vi "Dynamic Headers Change Headers.vi"(6 "Point Startup (WasherDOE)":path, 7 "Tree Selection":T2="1-1", 8 "Error In":errorcluster, 10 "Tool Base Path":path=path "C:/Technology Lab/NI-2010/Trunk/Refrigeration/RTS/Old System", 11 "Chamber Data":string[][](array[string])=[["System Date", "System Time", "Elapsed Time (sec)", "Elapsed Time (hrs)", "Voltage (V)", "RMS Current (Amps)", "Power (Watts)", "Watt Hours (Wh)", "Voltage Total Harmonic Distortion (%)", "Frequency (Hz)", "Apparent Power (VA)", "Power Factor", "TC 1", "TC 2", "TC 3", "TC 4", "TC 5", "TC 6", "TC 7", "TC 8", "TC 9", "TC 10", "TC 11", "TC 12", "TC 13", "TC 14", "TC 15", "TC 16", "TC 17", "TC 18", "TC 19", "TC 20", "TC 21", "TC 22", "TC 23", "TC 24", "TC 25", "TC 26", "TC 27", "TC 28", "TC 29", "TC 30", "AUX 1", "AUX 2", "CAL CL", "Room Setpoint Temperature", "Room Setpoint Humidity", "Room Temperature (°F)", "Room Humidity (%)", "Door Enable", "Room Setpoint Cool Temperature", "Room Setpoint Dehumidification Temperature", "Supply Temperature (°F)", "Cool Temperature (°F)", "Dehumidification Temperature (°F)", "Glycol Temperature (°F)", "Heat Rate (%)", "Steam Rate (%)", "Cool Rate (%)", "Dehumidification Rate (%)", "Room Status", "Room Dry P", "Room Dry I", "Room Humidity P", "Room Humidity I", "Room Heat P", "Room Heat I", "Room Cool Temperature P", "Room Cool Temperature I", "Room Dehumidification Temperature P", "Room Dehumidification Temperature I", "Voltage Setpoint 1", "60 Hz Power", "50 Hz Power", "120V Range", "240V Range", "Ground Line", "Ground Neutral", "Measure Ground Leakage Current", "Room OK", "S1 Freezer Relay", "S1 Cab Relay", "S1 Slide Relay", "Recording Data", "CVS Location", "Point Location"], ["01/24/2018", "06:36:24.375", "0.000000", "0.000000", "115.046623", "0.030182", "0.135573", "964.507616", "3.000000", "60.021709", "3.472371", "1.000000", "-2.310000", "-1.920000", "-0.910000", "327.670000", "327.670000", "327.670000", "327.670000", "327.670000", "327.670000", "327.670000", "38.020000", "35.660000", "35.030000", "327.670000", "327.670000", "327.670000", "327.670000", "327.670000", "327.670000", "327.670000", "327.670000", "327.670000", "327.670000", "70.360000", "327.670000", "327.670000", "70.300000", "327.670000", "32767.000000", "32767.000000", "0.001000", "0.000000", "1.988000", "70.000000", "35.000000", "70.040000", "38.150000", "1.000000", "55.000000", "48.000000", "66.700000", "55.180000", "48.160000", "0.000000", "36.920000", "0.000000", "30.630000", "8.240000", "0.000000", "200.000000", "15000.000000", "400.000000", "15000.000000", "1000.000000", "2000.000000", "500.000000", "6000.000000", "500.000000", "6000.000000", "115.000000", "1.000000", "0.000000", "1.000000", "0.000000", "0.000000", "1.000000", "0.000000", "1.000000", "0.000000", "0.000000", "0.000000", "FALSE", "", ""], ["System Date", "System Time", "Elapsed Time (sec)", "Elapsed Time (hrs)", "Voltage (V)", "RMS Current (Amps)", "Power (Watts)", "Watt Hours (Wh)", "Voltage Total Harmonic Distortion (%)", "Frequency (Hz)", "Apparent Power (VA)", "Power Factor", "TC 1", "TC 2", "TC 3", "TC 4", "TC 5", "TC 6", "TC 7", "TC 8", "TC 9", "TC 10", "TC 11", "TC 12", "TC 13", "TC 14", "TC 15", "TC 16", "TC 17", "TC 18", "TC 19", "TC 20", "TC 21", "TC 22", "TC 23", "TC 24", "TC 25", "TC 26", "TC 27", "TC 28", "TC 29", "TC 30", "AUX 1", "AUX 2", "CAL CL", "Room Setpoint Temperature", "Room Setpoint Humidity", "Room Temperature (°F)", "Room Humidity (%)", "Door Enable", "Room Setpoint Cool Temperature", "Room Setpoint Dehumidification Temperature", "Supply Temperature (°F)", "Cool Temperature (°F)", "Dehumidification Temperature (°F)", "Glycol Temperature (°F)", "Heat Rate (%)", "Steam Rate (%)", "Cool Rate (%)", "Dehumidification Rate (%)", "Room Status", "Room Dry P", "Room Dry I", "Room Humidity P", "Room Humidity I", "Room Heat P", "Room Heat I", "Room Cool Temperature P", "Room Cool Temperature I", "Room Dehumidification Temperature P", "Room Dehumidification Temperature I", "Voltage Setpoint 2", "60 Hz Power", "50 Hz Power", "120V Range", "240V Range", "Ground Line", "Ground Neutral", "Measure Ground Leakage Current", "Fault", "S2 Freezer Relay", "S2 Cab Relay", "S2 Slide Relay", "Recording Data", "CVS Location", "Point Location"], ["01/24/2018", "06:36:24.375", "0.000000", "0.000000", "114.863785", "0.030740", "0.139474", "26203.680290", "3.500000", "60.021633", "3.530865", "1.000000", "10.000000", "8.600000", "8.210000", "327.670000", "327.670000", "327.670000", "327.670000", "327.670000", "327.670000", "327.670000", "41.900000", "42.090000", "43.130000", "327.670000", "327.670000", "327.670000", "327.670000", "327.670000", "327.670000", "327.670000", "327.670000", "327.670000", "327.670000", "69.920000", "327.670000", "327.670000", "70.410000", "327.670000", "32767.000000", "32767.000000", "0.001000", "0.001000", "1.991000", "70.000000", "35.000000", "70.040000", "38.150000", "1.000000", "55.000000", "48.000000", "66.700000", "55.180000", "48.160000", "0.000000", "36.920000", "0.000000", "30.630000", "8.240000", "0.000000", "200.000000", "15000.000000", "400.000000", "15000.000000", "1000.000000", "2000.000000", "500.000000", "6000.000000", "500.000000", "6000.000000", "115.000000", "1.000000", "0.000000", "1.000000", "0.000000", "0.000000", "1.000000", "0.000000", "0.000000", "0.000000", "0.000000", "0.000000", "FALSE", "", ""], ["System Date", "System Time", "Elapsed Time (sec)", "Elapsed Time (hrs)", "Voltage (V)", "RMS Current (Amps)", "Power (Watts)", "Watt Hours (Wh)", "Voltage Total Harmonic Distortion (%)", "Frequency (Hz)", "Apparent Power (VA)", "Power Factor", "TC 1", "TC 2", "TC 3", "TC 4", "TC 5", "TC 6", "TC 7", "TC 8", "TC 9", "TC 10", "TC 11", "TC 12", "TC 13", "TC 14", "TC 15", "TC 16", "TC 17", "TC 18", "TC 19", "TC 20", "TC 21", "TC 22", "TC 23", "TC 24", "TC 25", "TC 26", "TC 27", "TC 28", "TC 29", "TC 30", "AUX 1", "AUX 2", "CAL CL", "Room Setpoint Temperature", "Room Setpoint Humidity", "Room Temperature (°F)", "Room Humidity (%)", "Door Enable", "Room Setpoint Cool Temperature", "Room Setpoint Dehumidification Temperature", "Supply Temperature (°F)", "Cool Temperature (°F)", "Dehumidification Temperature (°F)", "Glycol Temperature (°F)", "Heat Rate (%)", "Steam Rate (%)", "Cool Rate (%)", "Dehumidification Rate (%)", "Room Status", "Room Dry P", "Room Dry I", "Room Humidity P", "Room Humidity I", "Room Heat P", "Room Heat I", "Room Cool Temperature P", "Room Cool Temperature I", "Room Dehumidification Temperature P", "Room Dehumidification Temperature I", "Voltage Setpoint 3", "60 Hz Power", "50 Hz Power", "120V Range", "240V Range", "Ground Line", "Ground Neutral", "Measure Ground Leakage Current", "Room Heat", "S3 Freezer Relay", "S3 Cab Relay", "S3 Slide Relay", "Recording Data", "CVS Location", "Point Location"], ["01/24/2018", "06:36:24.376", "0.000000", "0.000000", "114.844543", "0.030078", "0.135316", "27955.201782", "3.100000", "60.022556", "3.456682", "1.000000", "0.690000", "0.850000", "2.060000", "327.670000", "327.670000", "327.670000", "327.670000", "327.670000", "327.670000", "327.670000", "37.750000", "38.160000", "38.080000", "327.670000", "327.670000", "327.670000", "327.670000", "327.670000", "327.670000", "327.670000", "327.670000", "327.670000", "327.670000", "70.410000", "327.670000", "327.670000", "70.770000", "327.670000", "32767.000000", "32767.000000", "0.001000", "0.001000", "1.963000", "70.000000", "35.000000", "70.040000", "38.150000", "1.000000", "55.000000", "48.000000", "66.700000", "55.180000", "48.160000", "0.000000", "36.920000", "0.000000", "30.630000", "8.240000", "0.000000", "200.000000", "15000.000000", "400.000000", "15000.000000", "1000.000000", "2000.000000", "500.000000", "6000.000000", "500.000000", "6000.000000", "115.000000", "1.000000", "0.000000", "1.000000", "0.000000", "0.000000", "1.000000", "0.000000", "1.000000", "0.000000", "0.000000", "0.000000", "FALSE", "", ""], ["System Date", "System Time", "Elapsed Time (sec)", "Elapsed Time (hrs)", "Voltage (V)", "RMS Current (Amps)", "Power (Watts)", "Watt Hours (Wh)", "Voltage Total Harmonic Distortion (%)", "Frequency (Hz)", "Apparent Power (VA)", "Power Factor", "TC 1", "TC 2", "TC 3", "TC 4", "TC 5", "TC 6", "TC 7", "TC 8", "TC 9", "TC 10", "TC 11", "TC 12", "TC 13", "TC 14", "TC 15", "TC 16", "TC 17", "TC 18", "TC 19", "TC 20", "TC 21", "TC 22", "TC 23", "TC 24", "TC 25", "TC 26", "TC 27", "TC 28", "TC 29", "TC 30", "AUX 1", "AUX 2", "CAL CL", "Room Setpoint Temperature", "Room Setpoint Humidity", "Room Temperature (°F)", "Room Humidity (%)", "Door Enable", "Room Setpoint Cool Temperature", "Room Setpoint Dehumidification Temperature", "Supply Temperature (°F)", "Cool Temperature (°F)", "Dehumidification Temperature (°F)", "Glycol Temperature (°F)", "Heat Rate (%)", "Steam Rate (%)", "Cool Rate (%)", "Dehumidification Rate (%)", "Room Status", "Room Dry P", "Room Dry I", "Room Humidity P", "Room Humidity I", "Room Heat P", "Room Heat I", "Room Cool Temperature P", "Room Cool Temperature I", "Room Dehumidification Temperature P", "Room Dehumidification Temperature I", "Voltage Setpoint 4", "60 Hz Power", "50 Hz Power", "120V Range", "240V Range", "Ground Line", "Ground Neutral", "Measure Ground Leakage Current", "Room Blower", "S4 Freezer Relay", "S4 Cab Relay", "S4 Slide Relay", "Recording Data", "CVS Location", "Point Location"], ["01/24/2018", "06:36:24.376", "0.000000", "0.000000", "115.200577", "0.030417", "0.136655", "26339.492026", "3.200000", "60.021862", "3.504017", "1.000000", "1.700000", "3.490000", "4.180000", "327.670000", "327.670000", "327.670000", "327.670000", "327.670000", "327.670000", "327.670000", "38.630000", "39.700000", "39.970000", "327.670000", "327.670000", "327.670000", "327.670000", "327.670000", "327.670000", "327.670000", "327.670000", "327.670000", "327.670000", "70.410000", "327.670000", "327.670000", "70.880000", "327.670000", "32767.000000", "32767.000000", "0.001000", "0.000000", "2.005000", "70.000000", "35.000000", "70.040000", "38.150000", "1.000000", "55.000000", "48.000000", "66.700000", "55.180000", "48.160000", "0.000000", "36.920000", "0.000000", "30.630000", "8.240000", "0.000000", "200.000000", "15000.000000", "400.000000", "15000.000000", "1000.000000", "2000.000000", "500.000000", "6000.000000", "500.000000", "6000.000000", "115.000000", "1.000000", "0.000000", "1.000000", "0.000000", "0.000000", "1.000000", "0.000000", "1.000000", "0.000000", "0.000000", "0.000000", "FALSE", "", ""], ["System Date", "System Time", "Elapsed Time (sec)", "Elapsed Time (hrs)", "Voltage (V)", "RMS Current (Amps)", "Power (Watts)", "Watt Hours (Wh)", "Voltage Total Harmonic Distortion (%)", "Frequency (Hz)", "Apparent Power (VA)", "Power Factor", "TC 1", "TC 2", "TC 3", "TC 4", "TC 5", "TC 6", "TC 7", "TC 8", "TC 9", "TC 10", "TC 11", "TC 12", "TC 13", "TC 14", "TC 15", "TC 16", "TC 17", "TC 18", "TC 19", "TC 20", "TC 21", "TC 22", "TC 23", "TC 24", "TC 25", "TC 26", "TC 27", "TC 28", "TC 29", "TC 30", "AUX 1", "AUX 2", "CAL CL", "Room Setpoint Temperature", "Room Setpoint Humidity", "Room Temperature (°F)", "Room Humidity (%)", "Door Enable", "Room Setpoint Cool Temperature", "Room Setpoint Dehumidification Temperature", "Supply Temperature (°F)", "Cool Temperature (°F)", "Dehumidification Temperature (°F)", "Glycol Temperature (°F)", "Heat Rate (%)", "Steam Rate (%)", "Cool Rate (%)", "Dehumidification Rate (%)", "Room Status", "Room Dry P", "Room Dry I", "Room Humidity P", "Room Humidity I", "Room Heat P", "Room Heat I", "Room Cool Temperature P", "Room Cool Temperature I", "Room Dehumidification Temperature P", "Room Dehumidification Temperature I", "Voltage Setpoint 5", "60 Hz Power", "50 Hz Power", "120V Range", "240V Range", "Ground Line", "Ground Neutral", "Measure Ground Leakage Current", "Spare", "S5 Freezer Relay", "S5 Cab Relay", "S5 Slide Relay", "Recording Data", "CVS Location", "Point Location"], ["01/24/2018", "06:36:24.376", "0.000000", "0.000000", "115.123596", "0.000000", "0.000000", "0.000000", "3.300000", "60.022747", "0.000000", "1.000000", "327.670000", "327.670000", "70.410000", "327.670000", "327.670000", "327.670000", "327.670000", "327.670000", "327.670000", "327.670000", "70.630000", "70.360000", "70.360000", "327.670000", "327.670000", "327.670000", "327.670000", "327.670000", "327.670000", "327.670000", "327.670000", "327.670000", "327.670000", "69.950000", "327.670000", "327.670000", "327.670000", "327.670000", "32767.000000", "32767.000000", "0.001000", "0.001000", "1.999000", "70.000000", "35.000000", "70.040000", "38.150000", "1.000000", "55.000000", "48.000000", "66.700000", "55.180000", "48.160000", "0.000000", "36.920000", "0.000000", "30.630000", "8.240000", "0.000000", "200.000000", "15000.000000", "400.000000", "15000.000000", "1000.000000", "2000.000000", "500.000000", "6000.000000", "500.000000", "6000.000000", "115.000000", "1.000000", "0.000000", "1.000000", "0.000000", "0.000000", "1.000000", "0.000000", "0.000000", "0.000000", "0.000000", "0.000000", "FALSE", "", ""], ["System Date", "System Time", "Elapsed Time (sec)", "Elapsed Time (hrs)", "Voltage (V)", "RMS Current (Amps)", "Power (Watts)", "Watt Hours (Wh)", "Voltage Total Harmonic Distortion (%)", "Frequency (Hz)", "Apparent Power (VA)", "Power Factor", "TC 1", "TC 2", "TC 3", "TC 4", "TC 5", "TC 6", "TC 7", "TC 8", "TC 9", "TC 10", "TC 11", "TC 12", "TC 13", "TC 14", "TC 15", "TC 16", "TC 17", "TC 18", "TC 19", "TC 20", "TC 21", "TC 22", "TC 23", "TC 24", "TC 25", "TC 26", "TC 27", "TC 28", "TC 29", "TC 30", "AUX 1", "AUX 2", "CAL CL", "Room Setpoint Temperature", "Room Setpoint Humidity", "Room Temperature (°F)", "Room Humidity (%)", "Door Enable", "Room Setpoint Cool Temperature", "Room Setpoint Dehumidification Temperature", "Supply Temperature (°F)", "Cool Temperature (°F)", "Dehumidification Temperature (°F)", "Glycol Temperature (°F)", "Heat Rate (%)", "Steam Rate (%)", "Cool Rate (%)", "Dehumidification Rate (%)", "Room Status", "Room Dry P", "Room Dry I", "Room Humidity P", "Room Humidity I", "Room Heat P", "Room Heat I", "Room Cool Temperature P", "Room Cool Temperature I", "Room Dehumidification Temperature P", "Room Dehumidification Temperature I", "Voltage Setpoint 6", "60 Hz Power", "50 Hz Power", "120V Range", "240V Range", "Ground Line", "Ground Neutral", "Measure Ground Leakage Current", "Room Pump", "S6 Freezer Relay", "S6 Cab Relay", "S6 Slide Relay", "Recording Data", "CVS Location", "Point Location"], ["01/24/2018", "06:36:24.376", "0.000000", "0.000000", "114.825302", "0.000000", "0.000000", "0.000000", "3.400000", "60.022854", "0.000000", "1.000000", "327.670000", "327.670000", "327.670000", "327.670000", "327.670000", "327.670000", "327.670000", "327.670000", "327.670000", "327.670000", "327.670000", "327.670000", "327.670000", "327.670000", "327.670000", "327.670000", "327.670000", "327.670000", "327.670000", "327.670000", "327.670000", "327.670000", "327.670000", "327.670000", "327.670000", "327.670000", "327.670000", "327.670000", "32767.000000", "32767.000000", "0.001000", "0.001000", "1.995000", "70.000000", "35.000000", "70.040000", "38.150000", "1.000000", "55.000000", "48.000000", "66.700000", "55.180000", "48.160000", "0.000000", "36.920000", "0.000000", "30.630000", "8.240000", "0.000000", "200.000000", "15000.000000", "400.000000", "15000.000000", "1000.000000", "2000.000000", "500.000000", "6000.000000", "500.000000", "6000.000000", "115.000000", "1.000000", "0.000000", "1.000000", "0.000000", "0.000000", "1.000000", "0.000000", "1.000000", "0.000000", "0.000000", "0.000000", "FALSE", "", ""], ["System Date", "System Time", "Elapsed Time (sec)", "Elapsed Time (hrs)", "Voltage (V)", "RMS Current (Amps)", "Power (Watts)", "Watt Hours (Wh)", "Voltage Total Harmonic Distortion (%)", "Frequency (Hz)", "Apparent Power (VA)", "Power Factor", "TC 1", "TC 2", "TC 3", "TC 4", "TC 5", "TC 6", "TC 7", "TC 8", "TC 9", "TC 10", "TC 11", "TC 12", "TC 13", "TC 14", "TC 15", "TC 16", "TC 17", "TC 18", "TC 19", "TC 20", "TC 21", "TC 22", "TC 23", "TC 24", "TC 25", "TC 26", "TC 27", "TC 28", "TC 29", "TC 30", "AUX 1", "AUX 2", "CAL CL", "Room Setpoint Temperature", "Room Setpoint Humidity", "Room Temperature (°F)", "Room Humidity (%)", "Door Enable", "Room Setpoint Cool Temperature", "Room Setpoint Dehumidification Temperature", "Supply Temperature (°F)", "Cool Temperature (°F)", "Dehumidification Temperature (°F)", "Glycol Temperature (°F)", "Heat Rate (%)", "Steam Rate (%)", "Cool Rate (%)", "Dehumidification Rate (%)", "Room Status", "Room Dry P", "Room Dry I", "Room Humidity P", "Room Humidity I", "Room Heat P", "Room Heat I", "Room Cool Temperature P", "Room Cool Temperature I", "Room Dehumidification Temperature P", "Room Dehumidification Temperature I", "Voltage Setpoint 7", "60 Hz Power", "50 Hz Power", "120V Range", "240V Range", "Ground Line", "Ground Neutral", "Measure Ground Leakage Current", "Spare", "S7 Freezer Relay", "S7 Cab Relay", "S7 Slide Relay", "Recording Data", "CVS Location", "Point Location"], ["01/24/2018", "06:36:24.376", "0.000000", "0.000000", "114.796432", "0.000000", "0.000000", "0.000000", "3.500000", "60.023220", "0.000000", "1.000000", "70.630000", "70.630000", "70.630000", "327.670000", "327.670000", "327.670000", "327.670000", "327.670000", "327.670000", "327.670000", "327.670000", "70.300000", "70.300000", "327.670000", "327.670000", "327.670000", "327.670000", "327.670000", "327.670000", "327.670000", "327.670000", "327.670000", "327.670000", "327.670000", "327.670000", "327.670000", "327.670000", "327.670000", "32767.000000", "32767.000000", "0.000000", "0.000000", "2.003000", "70.000000", "35.000000", "70.040000", "38.150000", "1.000000", "55.000000", "48.000000", "66.700000", "55.180000", "48.160000", "0.000000", "36.920000", "0.000000", "30.630000", "8.240000", "0.000000", "200.000000", "15000.000000", "400.000000", "15000.000000", "1000.000000", "2000.000000", "500.000000", "6000.000000", "500.000000", "6000.000000", "115.000000", "1.000000", "0.000000", "1.000000", "0.000000", "0.000000", "1.000000", "0.000000", "0.000000", "0.000000", "0.000000", "0.000000", "FALSE", "", ""], ["System Date", "System Time", "Elapsed Time (sec)", "Elapsed Time (hrs)", "Voltage (V)", "RMS Current (Amps)", "Power (Watts)", "Watt Hours (Wh)", "Voltage Total Harmonic Distortion (%)", "Frequency (Hz)", "Apparent Power (VA)", "Power Factor", "TC 1", "TC 2", "TC 3", "TC 4", "TC 5", "TC 6", "TC 7", "TC 8", "TC 9", "TC 10", "TC 11", "TC 12", "TC 13", "TC 14", "TC 15", "TC 16", "TC 17", "TC 18", "TC 19", "TC 20", "TC 21", "TC 22", "TC 23", "TC 24", "TC 25", "TC 26", "TC 27", "TC 28", "TC 29", "TC 30", "AUX 1", "AUX 2", "CAL CL", "Room Setpoint Temperature", "Room Setpoint Humidity", "Room Temperature (°F)", "Room Humidity (%)", "Door Enable", "Room Setpoint Cool Temperature", "Room Setpoint Dehumidification Temperature", "Supply Temperature (°F)", "Cool Temperature (°F)", "Dehumidification Temperature (°F)", "Glycol Temperature (°F)", "Heat Rate (%)", "Steam Rate (%)", "Cool Rate (%)", "Dehumidification Rate (%)", "Room Status", "Room Dry P", "Room Dry I", "Room Humidity P", "Room Humidity I", "Room Heat P", "Room Heat I", "Room Cool Temperature P", "Room Cool Temperature I", "Room Dehumidification Temperature P", "Room Dehumidification Temperature I", "Voltage Setpoint 8", "60 Hz Power", "50 Hz Power", "120V Range", "240V Range", "Ground Line", "Ground Neutral", "Measure Ground Leakage Current", "Spare", "S8 Freezer Relay", "S8 Cab Relay", "S8 Slide Relay", "Recording Data", "CVS Location", "Point Location"], ["01/24/2018", "06:36:24.377", "0.000000", "0.000000", "115.306419", "0.000000", "0.000000", "0.000000", "3.500000", "60.021893", "0.000000", "1.000000", "70.630000", "70.440000", "70.490000", "327.670000", "327.670000", "327.670000", "327.670000", "327.670000", "327.670000", "327.670000", "70.630000", "70.410000", "70.300000", "327.670000", "327.670000", "327.670000", "327.670000", "327.670000", "327.670000", "327.670000", "327.670000", "327.670000", "327.670000", "327.670000", "327.670000", "327.670000", "327.670000", "327.670000", "32767.000000", "32767.000000", "0.000000", "0.000000", "1.955000", "70.000000", "35.000000", "70.040000", "38.150000", "1.000000", "55.000000", "48.000000", "66.700000", "55.180000", "48.160000", "0.000000", "36.920000", "0.000000", "30.630000", "8.240000", "0.000000", "200.000000", "15000.000000", "400.000000", "15000.000000", "1000.000000", "2000.000000", "500.000000", "6000.000000", "500.000000", "6000.000000", "115.000000", "1.000000", "0.000000", "1.000000", "0.000000", "0.000000", "1.000000", "0.000000", "0.000000", "0.000000", "0.000000", "0.000000", "FALSE", "", ""]]) -> (0 "Error Out":errorcluster, 2 "Point File Path":path, 3 "New Header Save Array":T1[](array[typedef]), 5 "Default Headers":bool)   [LabVIEW 2018]
uses:
  Washer DOE/Type Definitions/DOE Data Save Modifier.ctl
  Refrigeration/RTS/Type Definitions/RTS Point File.ctl
  Refrigeration/RTS/Type Definitions/RTS Room Selector.ctl
panel:
  in  "Save Point File":bool
  in  "Delete Point File":bool
  in  "Header Save Array":T1[](array[typedef])
  in  "Point File Name":string(combo)
  in  "Use Default Headers":bool
  in  "Tab Control":enum32{"Page 1", "Page 2"}(tab)
  out "Point Data":T3[](array[typedef])
  in  "Debug":bool
  out "Debug States":string[](array[string])
  in  "Update Server":bool
  out "Front Program Name":string
  # "Name"
  # "Title"
  # "Group"
  # "Save Status"
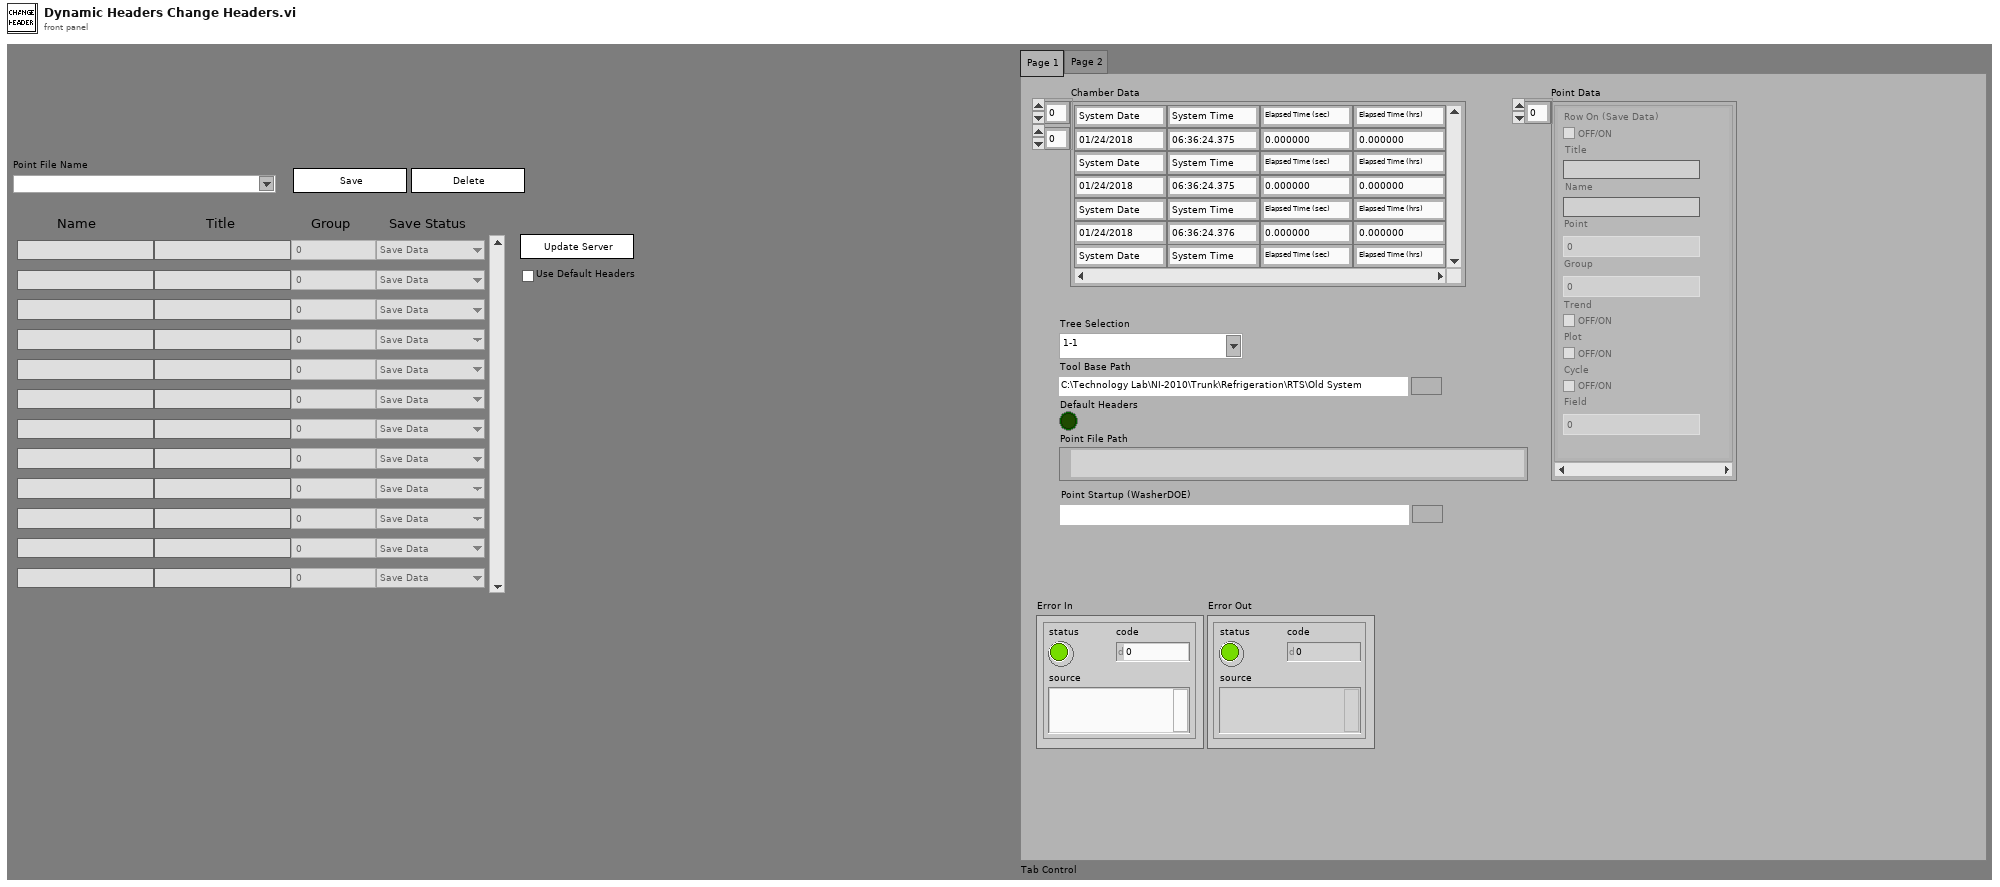
[diagram p1: front panel]
types:
  T1 = typedef "DOE Data Save Modifier.ctl" = cluster{"Name":string, "Title":string, "Save Status":enum16{"Save Data", "Don't Save Data"}, "Group":u8, "Field":u8}
  T2 = typedef "RTS Room Selector.ctl" = string
  T3 = typedef "RTS Point File.ctl" = cluster{"Title":string, "Name":string, "Point":u8, "Plot":bool, "Trend":bool, "Cycle":bool, "Field":u8, "Row On (Save Data)":bool, "Group":u8}
  T4 = enum32{"invalid app kind", "Development System", "Run Time System", "Student Edition", "Embedded LabVIEW", "Evaluation", "Custom"}
  T5 = enum32{"Invalid", "Standard", "Closed", "Hidden", "Minimized", "Maximized"}
  T6 = cluster{"Core":cluster{"Current VI Reference":refnum<vi>, "Close Panel on Exit?":bool}, "Default Headers":bool, "Header Save Array":T1[], "Chamber Data":string[][], "appended path":path, "Point Array":T3[], "Write Path":path, "Tree Selection":T2, "Point Startup (WasherDOE)":path}
  T7 = cluster{"Current VI Reference":refnum<vi>, "Close Panel on Exit?":bool}
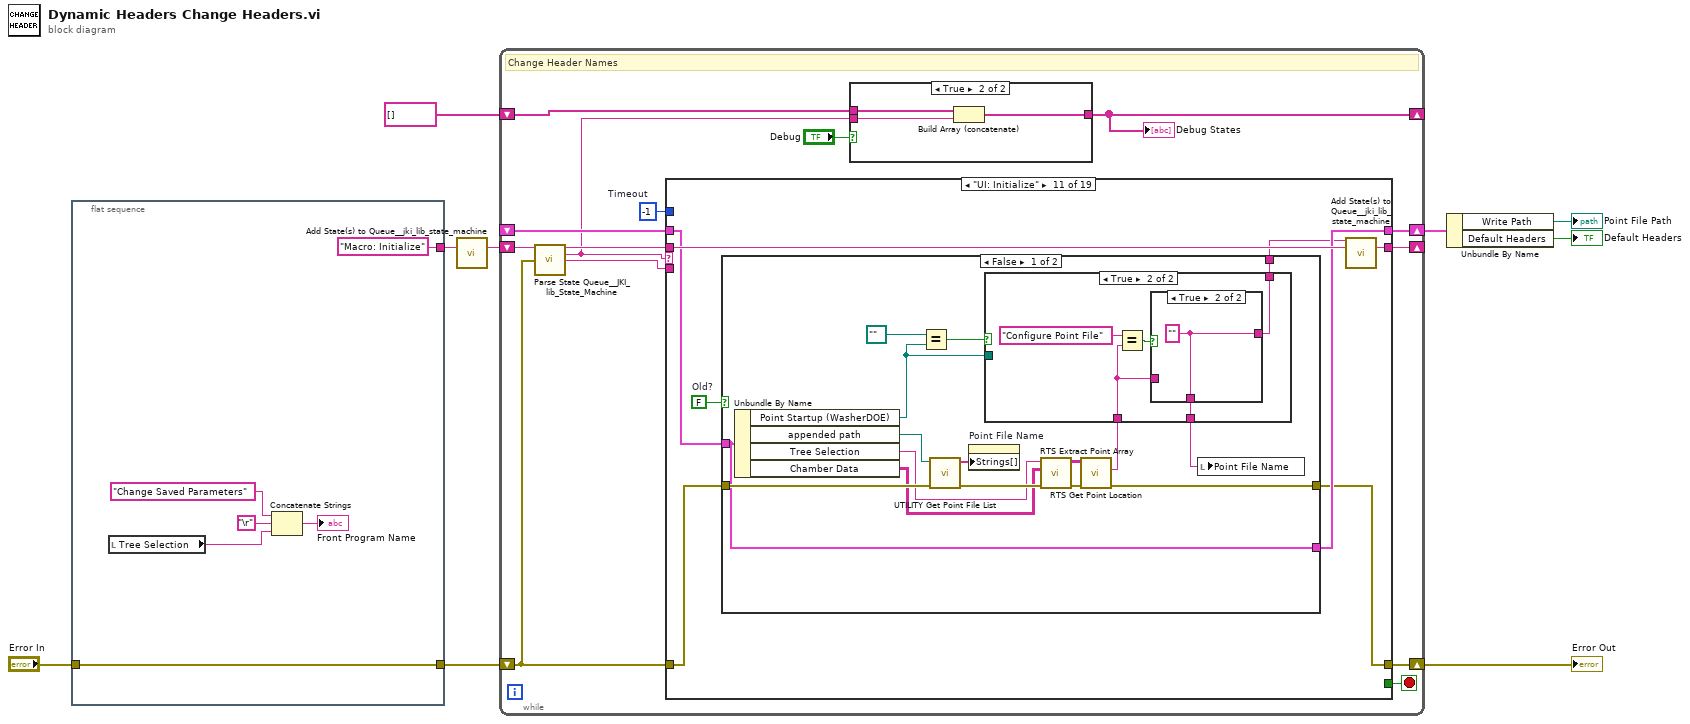
[diagram p0: block diagram]
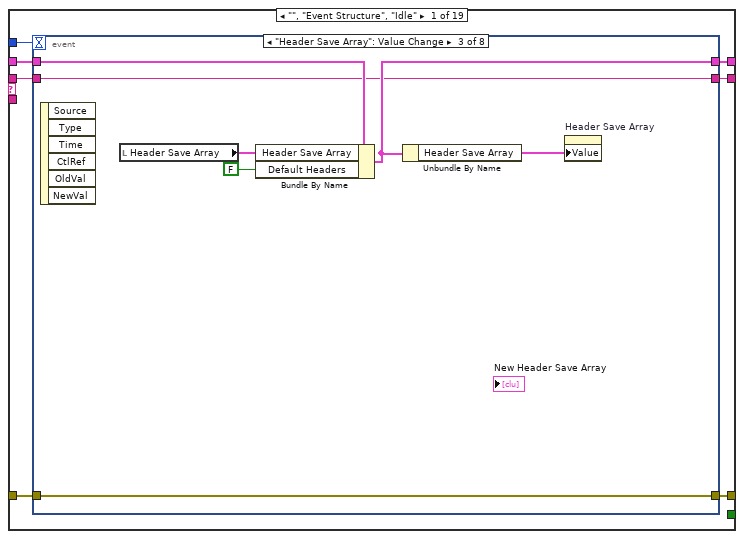
[diagram p3: hidden frame]
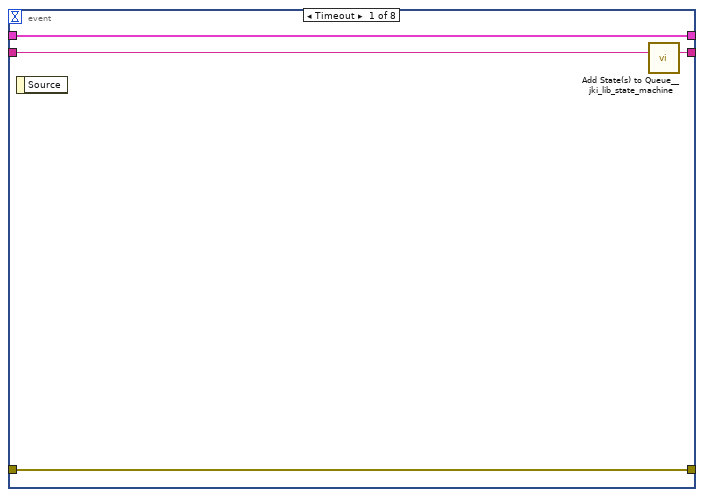
[diagram p4: hidden frame]
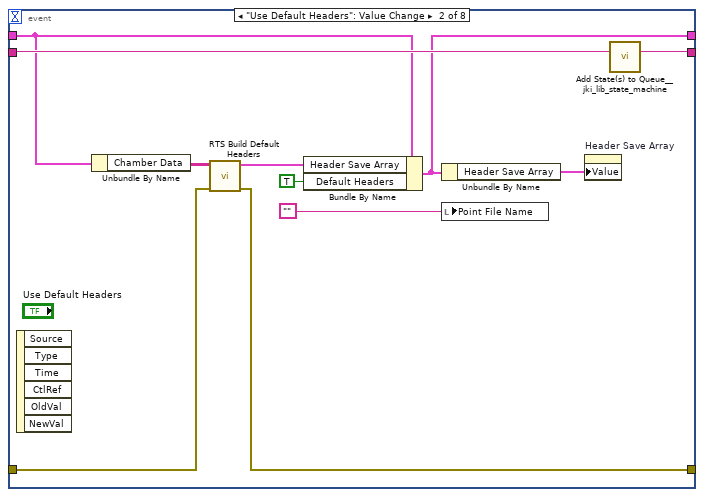
[diagram p5: hidden frame]
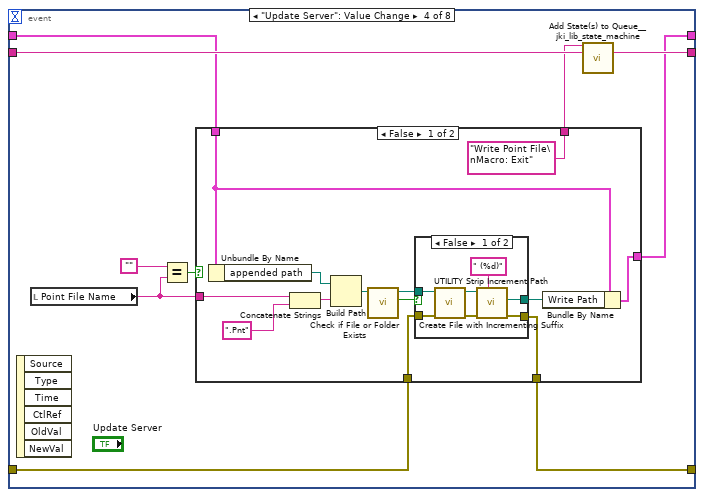
[diagram p6: hidden frame]
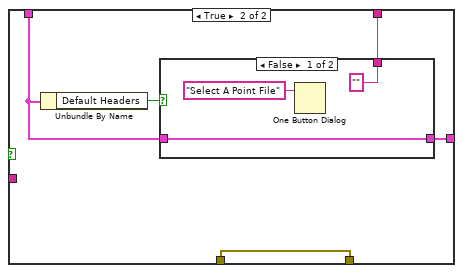
[diagram p8: hidden frame]
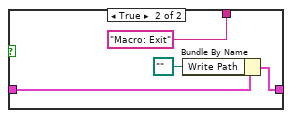
[diagram p9: hidden frame]
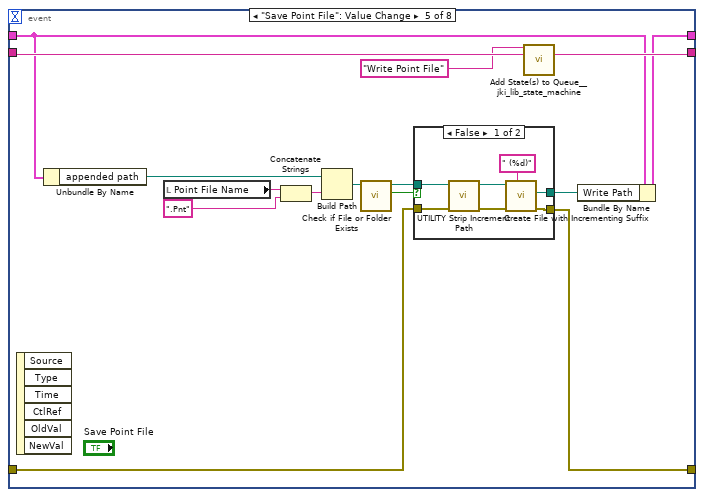
[diagram p10: hidden frame]
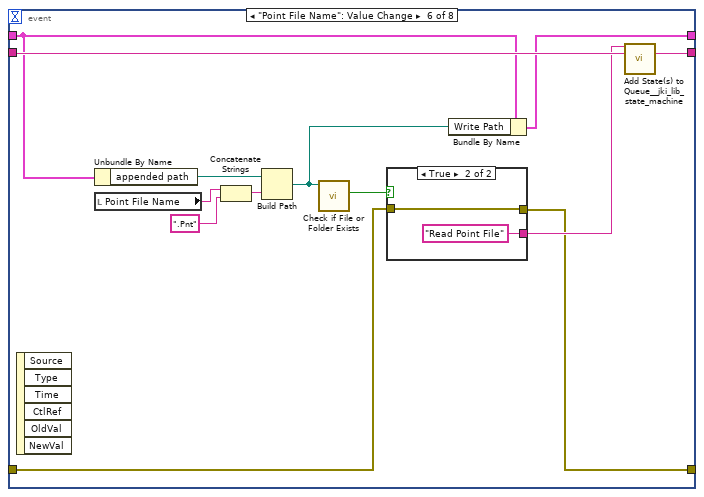
[diagram p12: hidden frame]
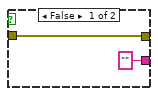
[diagram p13: hidden frame]
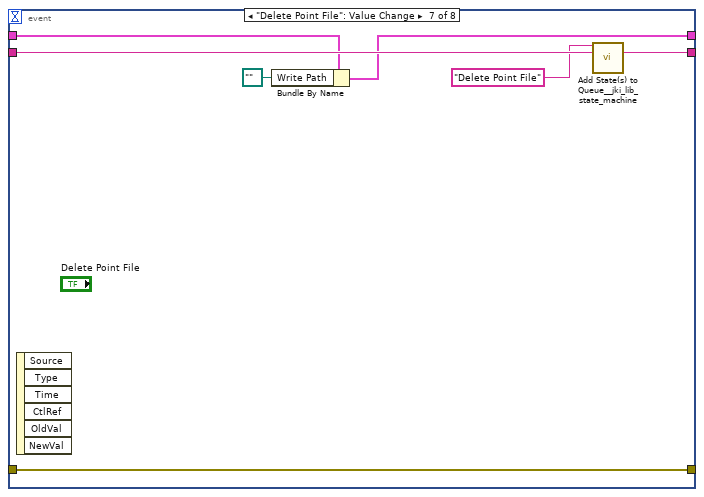
[diagram p14: hidden frame]
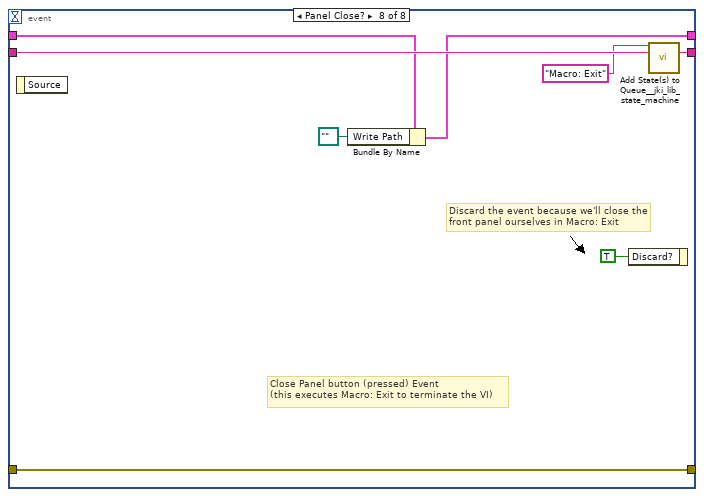
[diagram p15: hidden frame]
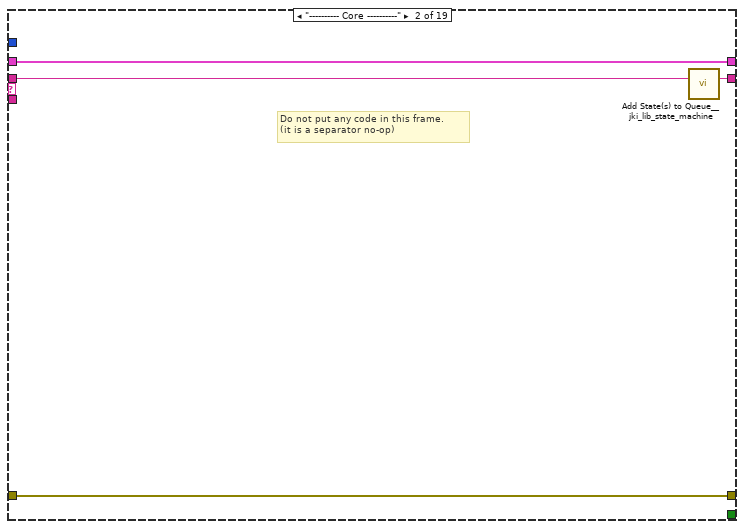
[diagram p16: hidden frame]
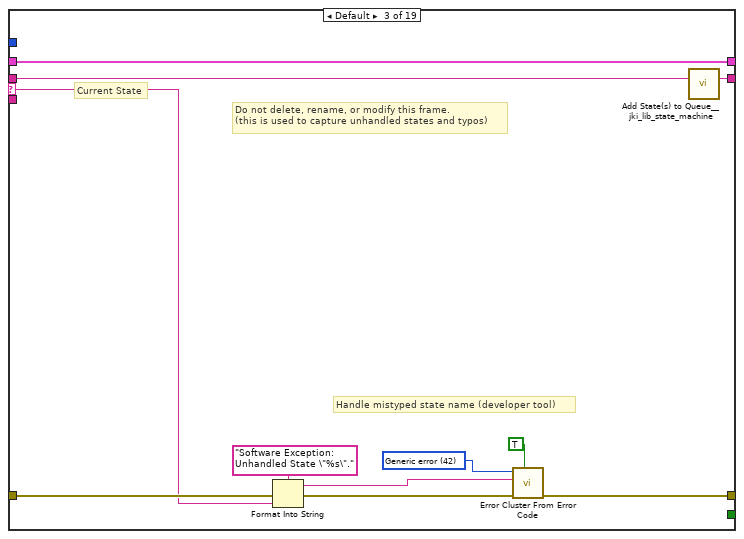
[diagram p17: hidden frame]
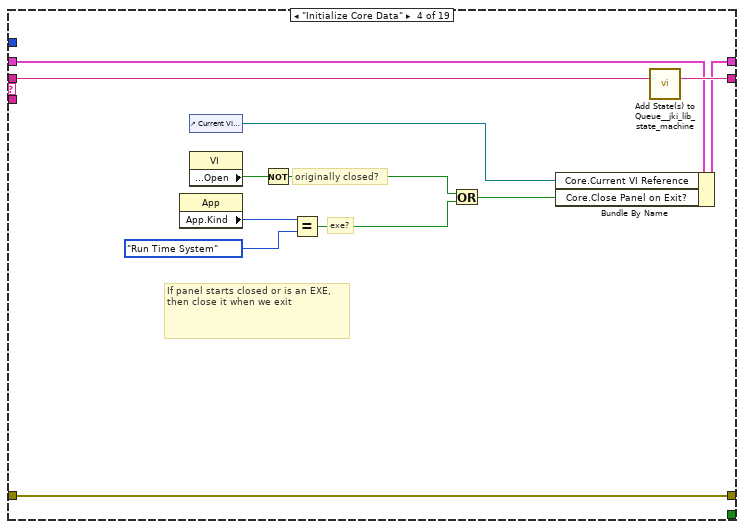
[diagram p18: hidden frame]
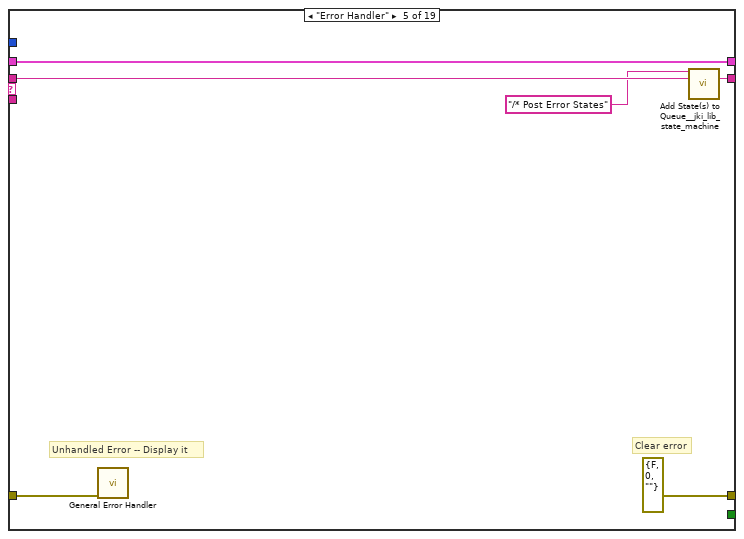
[diagram p19: hidden frame]
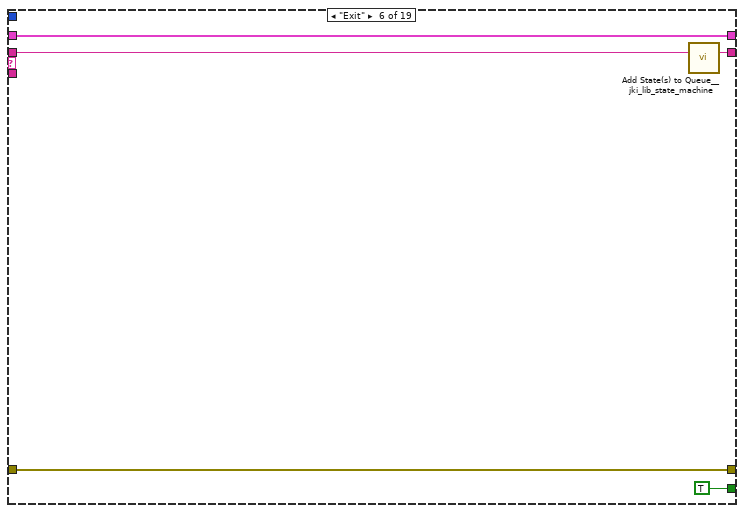
[diagram p20: hidden frame]
diagram:
  n1 = flat-sequence {
    tunnel: [w15] -> w6
    tunnel: "Error In" -> [w15]
    tunnel: ["Macro: Initialize"] -> w5
    frame #0 {
      n2 = local read "Tree Selection"() -> (w10:T2)
      n3 = Concatenate Strings("Change Saved Parameters" ("string"), "\r", w10) -> (→"Front Program Name":string)
    }
  }
  n4 = call <vilib>:"Add State(s) to Queue__jki_lib_state_machine.vi"("State(s) in (\"\")"=w5) -> ("States Out"=w9:string)  [unwired: 14 in]
  n5 = while "Change Header Names" {
    shift-right: [w23] -> w3
    shift-left: _ -> [w22]
    shift-right: [w26] -> w8
    shift-left: w6 -> [w20]
    shift-right: [w25] -> _
    shift-left: w9 -> [w27]
    shift-right: [w17] -> _
    shift-left: string[] [] -> [w19]
    stop <- w24 stop-if-true
    w21 = -1  # Timeout
    # "Change Header Names"
    n6 = call <vilib>:"Parse State Queue__JKI_lib_State_Machine.vi"("State Queue"=w27, "Error In (no error)"=w20) -> ("Remaining States"=w29:string, "Current State"=w18:string, "Arguments"=w28:string)  [unwired: 11 in]
    n7 = case shown="\"UI: Initialize\"" w18 {
      selector: w18 -> [_ _ w167 _ _ _ _ _ _ _ _ _ _ _ _ _ _ _ _]
      tunnel: w29 -> [w40 w166 w171 w189 w195 w200 w204 w219 w225 w229 w237 w278 w289 w315 w320 w340 w351 w366 w378]
      tunnel: w28 -> [_ _ _ _ _ _ _ _ _ _ _ w273 w283 _ _ _ _ _ _]
      tunnel: w22 -> [w38 w163 w169 w180 w192 w198 w201 _ w220 w226 w235 w276 w285 w312 w317 w333 w348 w364 w375]
      tunnel: [w37 w164 w173 w186 errorcluster {"status"=FALSE, "code"=0, "source"=""} ("error out") w197 w202 w216 w221 w227 w231 w274 w286 w313 w318 w334 w342 w352 w376] -> w26
      tunnel: w20 -> [w36 w164 w172 w186 w191 w197 w202 w216 w222 w227 w232 w275 w287 w313 w318 w337 w349 w359 w376]
      tunnel: [w39 w165 w170 w188 w194 w199 w203 w218 w224 w228 w236 w277 w288 w314 w319 w339 w350 w365 w377] -> w25
      tunnel: [_ _ _ _ _ TRUE _ _ _ _ _ _ _ _ _ _ _ _ _] -> w24
      tunnel: [w35 w163 w169 w187 w192 w198 w201 w217 w220 w226 w234 w276 w285 w312 w317 w332 w348 w364 w375] -> w23
      tunnel: w21 -> [w34 _ _ _ _ _ _ _ _ _ _ _ _ _ _ _ _ _ _]
      frame "", "Event Structure", "Idle" {
        n8 = event shown="[2] \"Header Save Array\": Value Change" {
          selector: _ -> [_ _ _ _ _ _ _ _]
          dyn-events: _ -> [_ _ _ _ _ _ _ _]
          timeout: w34 -> [_ _ _ _ _ _ _ _]
          tunnel: w40 -> [w44 w54 w58 w71 w120 w142 w152 w162]
          tunnel: [w43 w55 w58 w72 w121 w143 w153 w161] -> w39
          tunnel: w38 -> [w41 w51 w61 w66 w112 w133 w150 w157]
          tunnel: [w42 w48 w60 w68 w107 w134 w154 w160] -> w37
          tunnel: w36 -> [w42 w49 w60 w69 w113 w135 w154 w160]
          tunnel: [w41 w53 w59 w67 w111 w132 w149 w156] -> w35
          event Timeout {
            n9 = event-data() -> ()  [unwired: 1 in, 1 out]
            n10 = call <vilib>:"Add State(s) to Queue__jki_lib_state_machine.vi"("State(s) in (\"\")"=w44) -> ("States Out"=w43:string)  [unwired: 14 in]
          }
          event "Use Default Headers": Value Change {
            n11 = event-data() -> ()  [unwired: 1 in, 6 out]
            n12 = Unbundle By Name(w51) -> ("Chamber Data"=w50:string[][])
            n13 = call "RTS Build Default Headers.vi"("Error In"=w49, "Chamber Data in"=w50) -> ("Error Out"=w48:errorcluster, "New Header Save Array"=w47:T1[])  [unwired: 8 in]
            n14 = Bundle By Name(cluster=w51, "Header Save Array"=w47, "Default Headers"=TRUE) -> (w53:T6)
            n15 = Unbundle By Name(w53) -> ("Header Save Array"=w52:T1[])
            n16 = local write "Point File Name"("") -> ()
            n17 = property on="Header Save Array" class="Arr (strict)"("Value"=w52) -> ()  [unwired: 2 in, 2 out]
            n18 = call <vilib>:"Add State(s) to Queue__jki_lib_state_machine.vi"("State(s) in (\"\")"=w54) -> ("States Out"=w55:string)  [unwired: 14 in]
          }
          event "Header Save Array": Value Change {
            n19 = event-data() -> ()  [unwired: 1 in, 6 out]
            n20 = local read "Header Save Array"() -> (w62:T1[])
            n21 = Bundle By Name(cluster=w61, "Header Save Array"=w62, "Default Headers"=FALSE) -> (w59:T6)
            n22 = Unbundle By Name(w59) -> ("Header Save Array"=w57:T1[])
            n23 = property on="Header Save Array" class="Arr (strict)"("Value"=w57) -> ()  [unwired: 2 in, 2 out]
          }
          event "Update Server": Value Change {
            n24 = event-data() -> ()  [unwired: 1 in, 6 out]
            n25 = local read "Point File Name"() -> (w65:string)
            n26 = Equal?(x="", y=w65) -> (x = y?=w63:bool)
            n27 = case shown="False" w63 {
              tunnel: ["Write Point File\nMacro: Exit" w97] -> w70
              tunnel: w69 -> [w82 w99]
              tunnel: [w81 w99] -> w68
              tunnel: [w80 w95] -> w67
              tunnel: w66 -> [w79 w96]
              tunnel: w65 -> [w76 _]
              frame False {
                n28 = Unbundle By Name(w79) -> ("appended path"=w84:path)
                n29 = Concatenate Strings(w76, ".Pnt" ("pattern")) -> (w77:string)
                n30 = Build Path(base path=w84, name or relative path=w77) -> (appended path=w75:path)
                n31 = call <vilib>:"Check if File or Folder Exists.vi"("path"=w75) -> ("file or folder exists?"=w74:bool, "dup path"=w73:path)  [unwired: 8 in, 1 out]
                n32 = case shown="False" w74 {
                  tunnel: w73 -> [w86 w93]
                  tunnel: w82 -> [w89 w94]
                  tunnel: [w91 w94] -> w81
                  tunnel: [w90 w93] -> w83
                  frame False {
                    n33 = call "UTILITY Strip Increment Path.vi"("Error In"=w89, "file path in"=w86) -> ("Error Out"=w88:errorcluster, "file path out"=w87:path)  [unwired: 8 in]
                    n34 = call <vilib>:"Create File with Incrementing Suffix.vi"("format string (\" (%d)\")"=" (%d)" ("format string (\" (%d)\")"), "error in (no error)"=w88, "file path"=w87) -> ("error out"=w91:errorcluster, "actual path"=w90:path)  [unwired: 6 in, 1 out]
                  }
                  frame True {
                  }
                }
                n35 = Bundle By Name(cluster=w79, "Write Path"=w83) -> (w80:T6)
              }
              frame True {
                n36 = Unbundle By Name(w96) -> ("Default Headers"=w98:bool)
                n37 = case shown="False" w98 {
                  tunnel: ["" "Macro: Exit"] -> w97
                  tunnel: w96 -> [w100 w104]
                  tunnel: [w100 w103] -> w95
                  frame False {
                    n38 = One Button Dialog(message="Select A Point File") -> ()  [unwired: 1 in, 1 out]
                  }
                  frame True {
                    n39 = Bundle By Name(cluster=w104, "Write Path"=path "") -> (w103:T6)
                  }
                }
              }
            }
            n40 = call <vilib>:"Add State(s) to Queue__jki_lib_state_machine.vi"("State(s) in Front (\"\")"=w70, "State(s) in (\"\")"=w71) -> ("States Out"=w72:string)  [unwired: 13 in]
          }
          event "Save Point File": Value Change {
            n41 = event-data() -> ()  [unwired: 1 in, 6 out]
            n42 = Unbundle By Name(w112) -> ("appended path"=w108:path)
            n43 = local read "Point File Name"() -> (w117:string)
            n44 = Concatenate Strings(w117, ".Pnt" ("pattern")) -> (w118:string)
            n45 = Build Path(base path=w108, name or relative path=w118) -> (appended path=w116:path)
            n46 = call <vilib>:"Check if File or Folder Exists.vi"("path"=w116) -> ("file or folder exists?"=w115:bool, "dup path"=w114:path)  [unwired: 8 in, 1 out]
            n47 = case shown="False" w115 {
              tunnel: w114 -> [w125 w129]
              tunnel: w113 -> [w123 w130]
              tunnel: [w127 w130] -> w107
              tunnel: [w126 w129] -> w110
              frame False {
                n48 = call "UTILITY Strip Increment Path.vi"("Error In"=w123, "file path in"=w125) -> ("Error Out"=w122:errorcluster, "file path out"=w124:path)  [unwired: 8 in]
                n49 = call <vilib>:"Create File with Incrementing Suffix.vi"("format string (\" (%d)\")"=" (%d)" ("format string (\" (%d)\")"), "error in (no error)"=w122, "file path"=w124) -> ("error out"=w127:errorcluster, "actual path"=w126:path)  [unwired: 6 in, 1 out]
              }
              frame True {
              }
            }
            n50 = call <vilib>:"Add State(s) to Queue__jki_lib_state_machine.vi"("State(s) in Front (\"\")"="Write Point File", "State(s) in (\"\")"=w120) -> ("States Out"=w121:string)  [unwired: 13 in]
            n51 = Bundle By Name(cluster=w112, "Write Path"=w110) -> (w111:T6)
          }
          event "Point File Name": Value Change {
            n52 = event-data() -> ()  [unwired: 1 in, 6 out]
            n53 = Unbundle By Name(w133) -> ("appended path"=w139:path)
            n54 = local read "Point File Name"() -> (w138:string)
            n55 = Concatenate Strings(w138, ".Pnt" ("pattern")) -> (w140:string)
            n56 = Build Path(base path=w139, name or relative path=w140) -> (appended path=w131:path)
            n57 = call <vilib>:"Check if File or Folder Exists.vi"("path"=w131) -> ("file or folder exists?"=w136:bool)  [unwired: 8 in, 2 out]
            n58 = case shown="True" w136 {
              tunnel: ["" "Read Point File"] -> w137
              tunnel: w135 -> [w144 w146]
              tunnel: [w144 w146] -> w134
              frame False {
              }
              frame True {
              }
            }
            n59 = Bundle By Name(cluster=w133, "Write Path"=w131) -> (w132:T6)
            n60 = call <vilib>:"Add State(s) to Queue__jki_lib_state_machine.vi"("State(s) in Front (\"\")"=w137, "State(s) in (\"\")"=w142) -> ("States Out"=w143:string)  [unwired: 13 in]
          }
          event "Delete Point File": Value Change {
            n61 = event-data() -> ()  [unwired: 1 in, 6 out]
            n62 = Bundle By Name(cluster=w150, "Write Path"=path "") -> (w149:T6)
            n63 = call <vilib>:"Add State(s) to Queue__jki_lib_state_machine.vi"("State(s) in Front (\"\")"="Delete Point File" ("State(s) in Front (\"\")"), "State(s) in (\"\")"=w152) -> ("States Out"=w153:string)  [unwired: 13 in]
          }
          event Panel Close? {
            # "Discard the event because we'll close the front panel ourselves in Macro: Exit"
            # "Close Panel button (pressed) Event\n(this executes Macro: Exit to terminate the VI)"
            n64 = event-data() -> ()  [unwired: 1 in, 1 out]
            n65 = Bundle By Name(cluster=w157, "Write Path"=path "") -> (w156:T6)
            n66 = event-data("Discard?"=TRUE) -> ()  [unwired: 1 in, 1 out]
            n67 = call <vilib>:"Add State(s) to Queue__jki_lib_state_machine.vi"("State(s) in Front (\"\")"="Macro: Exit", "State(s) in (\"\")"=w162) -> ("States Out"=w161:string)  [unwired: 13 in]
          }
        }
      }
      frame "---------- Core ----------" {
        # "Do not put any code in this frame.\n(it is a separator no-op)"
        n68 = call <vilib>:"Add State(s) to Queue__jki_lib_state_machine.vi"("State(s) in (\"\")"=w166) -> ("States Out"=w165:string)  [unwired: 14 in]
      }
      frame Default {
        w176 = 42 items=["No error", "Argument error", "Memory is full", "Out of zone", "End of file", "File already open", "Generic file I/O error", "File not found", "File permission error", "Disk is full", "Duplicate path", "Too many files open", "System feature not enabled", "Resource file not found", "Cannot add resource", "Resource not found", "Image not found", "Image memory error", "Pen does not exist", "Config type invalid", "Config token not found", "Config parse error", "Config memory error", "Bad external code format", "Bad external code offset", "External code not present", "Null window", "Destroy window error", "Null menu", "Print aborted", "Bad print record", "Print driver error", "Windows error during printing", "Memory error during printing", "Print dialog error", "Generic print error", "Invalid device refnum", "Device not found", "Device parameter error", "Device unit error", "Cannot open device", "Device call aborted", "Generic error", "Cancelled by user", "Object ID too low", "Object ID too high", "Object not in heap", "Unknown heap", "Unknown object (invalid DefProc)", "Unknown object (DefProc not in table)", "Message out of range", "Invalid (null) method", "Unknown message", "Manager call not supported", "Bad address", "Network operation in progress", "Network operation timed out", "Connection is busy", "Network attribute not supported", "Network error", "Address in use", "System out of memory", "Connection aborted", "Connection refused", "Not connected", "Already connected", "Connection closed", "Initialization error (interapplication manager)", "Bad occurrence", "Wait on unbound occurrence handler", "Occurrence queue overflow", "Datalog type conflict", "Unused", "Unrecognized type (interapplication manager)", "Memory corrupt", "Failed to make temporary DLL", "Old CIN version", "Drag socket not found", "Failed to load drop-object", "Failed to register OLE object", "Failed to release OLE object", "Format specifier type mismatch", "Unknown format specifier", "Too few format specifiers", "Too many format specifiers", "Scan failed", "Newer CIN version", "Error converting to variant", "Runtime menu error", "Password tampered", "Variant attribute not found", "Incompatible variant data type", "Event data is not available", "Event Store is not present", "Occurrence is not found", "Event Queue is not created", "Event info is not available", "Refnum passed is NULL", "Error retrieving Class GUID", "Error retrieving CoClass GUID", "Error retrieving TypeLib GUID.", "Bad built application magic bytes.", "Specific driver is different from the specific driver associated with the Logical Name.", "There is no session opened to the class driver.", "Max Error", "MAX - Error with config objects", "MAX - Error loading configuration", "MAX - Group not supported"]
        # "Current State"
        # "Do not delete, rename, or modify this frame.\n(this is used to capture unhandled states and typos)"
        # "Handle mistyped state name (developer tool)"
        n69 = Format Into String(format string="Software Exception: Unhandled State \"%s\"." ("message"), error in=w172, w167) -> (resulting string=w175:string, error out=w174:errorcluster)  [unwired: 1 in]
        n70 = call <vilib>:"Error Cluster From Error Code.vi"("show call chain? (False)"=TRUE, "error in (no error)"=w174, "error message (\"\")"=w175, "error code (0)"=w176) -> ("error out"=w173:errorcluster)  [unwired: 5 in]
        n71 = call <vilib>:"Add State(s) to Queue__jki_lib_state_machine.vi"("State(s) in (\"\")"=w171) -> ("States Out"=w170:string)  [unwired: 14 in]
      }
      frame "Initialize Core Data" {
        # "originally closed?"
        # "exe?"
        # "If panel starts closed or is an EXE, then close it when we exit"
        n72 = property class="App"() -> ("App.Kind"=w184:T4)  [unwired: 2 in, 2 out]
        n73 = control-ref of="Current VI Reference"() -> (w178:refnum<vi>)
        n74 = property class="VI"() -> ("Front Panel.Open"=w185:bool)  [unwired: 2 in, 2 out]
        n75 = Not(x=w185) -> (.not. x?=w182:bool)
        n76 = Equal?(x=w184, y=T4."Run Time System" ("Application:Kind")) -> (x = y?=w181:bool)
        n77 = Or(x=w182, y=w181) -> (x .or. y?=w179:bool)
        n78 = Bundle By Name(cluster=w180, "Core.Current VI Reference"=w178, "Core.Close Panel on Exit?"=w179) -> (w187:T6)
        n79 = call <vilib>:"Add State(s) to Queue__jki_lib_state_machine.vi"("State(s) in (\"\")"=w189) -> ("States Out"=w188:string)  [unwired: 14 in]
      }
      frame "Error Handler" {
        # "Unhandled Error -- Display it"
        # "Clear error"
        n80 = call <vilib>:"General Error Handler.vi"("error in (no error)"=w191) -> ()  [unwired: 10 in, 5 out]
        n81 = call <vilib>:"Add State(s) to Queue__jki_lib_state_machine.vi"("State(s) in Front (\"\")"="/* Post Error States", "State(s) in (\"\")"=w195) -> ("States Out"=w194:string)  [unwired: 13 in]
      }
      frame "Exit" {
        n82 = call <vilib>:"Add State(s) to Queue__jki_lib_state_machine.vi"("State(s) in (\"\")"=w200) -> ("States Out"=w199:string)  [unwired: 14 in]
      }
      frame "---------- Data ----------" {
        n83 = call <vilib>:"Add State(s) to Queue__jki_lib_state_machine.vi"("State(s) in (\"\")"=w204) -> ("States Out"=w203:string)  [unwired: 14 in]
      }
      frame "Data: Initialize" {
        w208 = path ""  # Write Path
        w209 = T3[] [{"Title"="", "Name"="", "Point"=0, "Plot"=FALSE, "Trend"=FALSE, "Cycle"=FALSE, "Field"=0, "Row On (Save Data)"=FALSE, "Group"=0}, {"Title"="", "Name"="", "Point"=0, "Plot"=FALSE, "Trend"=FALSE, "Cycle"=FALSE, "Field"=0, "Row On (Save Data)"=FALSE, "Group"=0}, {"Title"="", "Name"="", "Point"=0, "Plot"=FALSE, "Trend"=FALSE, "Cycle"=FALSE, "Field"=0, "Row On (Save Data)"=FALSE, "Group"=0}, {"Title"="", "Name"="", "Point"=0, "Plot"=FALSE, "Trend"=FALSE, "Cycle"=FALSE, "Field"=0, "Row On (Save Data)"=FALSE, "Group"=0}, {"Title"="", "Name"="", "Point"=0, "Plot"=FALSE, "Trend"=FALSE, "Cycle"=FALSE, "Field"=0, "Row On (Save Data)"=FALSE, "Group"=0}, {"Title"="", "Name"="", "Point"=0, "Plot"=FALSE, "Trend"=FALSE, "Cycle"=FALSE, "Field"=0, "Row On (Save Data)"=FALSE, "Group"=0}, {"Title"="", "Name"="", "Point"=0, "Plot"=FALSE, "Trend"=FALSE, "Cycle"=FALSE, "Field"=0, "Row On (Save Data)"=FALSE, "Group"=0}, {"Title"="", "Name"="", "Point"=0, "Plot"=FALSE, "Trend"=FALSE, "Cycle"=FALSE, "Field"=0, "Row On (Save Data)"=FALSE, "Group"=0}, {"Title"="", "Name"="", "Point"=0, "Plot"=FALSE, "Trend"=FALSE, "Cycle"=FALSE, "Field"=0, "Row On (Save Data)"=FALSE, "Group"=0}, {"Title"="", "Name"="", "Point"=0, "Plot"=FALSE, "Trend"=FALSE, "Cycle"=FALSE, "Field"=0, "Row On (Save Data)"=FALSE, "Group"=0}, {"Title"="", "Name"="", "Point"=0, "Plot"=FALSE, "Trend"=FALSE, "Cycle"=FALSE, "Field"=0, "Row On (Save Data)"=FALSE, "Group"=0}, {"Title"="", "Name"="", "Point"=0, "Plot"=FALSE, "Trend"=FALSE, "Cycle"=FALSE, "Field"=0, "Row On (Save Data)"=FALSE, "Group"=0}, {"Title"="", "Name"="", "Point"=0, "Plot"=FALSE, "Trend"=FALSE, "Cycle"=FALSE, "Field"=0, "Row On (Save Data)"=FALSE, "Group"=0}, {"Title"="", "Name"="", "Point"=0, "Plot"=FALSE, "Trend"=FALSE, "Cycle"=FALSE, "Field"=0, "Row On (Save Data)"=FALSE, "Group"=0}, {"Title"="", "Name"="", "Point"=0, "Plot"=FALSE, "Trend"=FALSE, "Cycle"=FALSE, "Field"=0, "Row On (Save Data)"=FALSE, "Group"=0}, {"Title"="", "Name"="", "Point"=0, "Plot"=FALSE, "Trend"=FALSE, "Cycle"=FALSE, "Field"=0, "Row On (Save Data)"=FALSE, "Group"=0}, {"Title"="", "Name"="", "Point"=0, "Plot"=FALSE, "Trend"=FALSE, "Cycle"=FALSE, "Field"=0, "Row On (Save Data)"=FALSE, "Group"=0}, {"Title"="", "Name"="", "Point"=0, "Plot"=FALSE, "Trend"=FALSE, "Cycle"=FALSE, "Field"=0, "Row On (Save Data)"=FALSE, "Group"=0}, {"Title"="", "Name"="", "Point"=0, "Plot"=FALSE, "Trend"=FALSE, "Cycle"=FALSE, "Field"=0, "Row On (Save Data)"=FALSE, "Group"=0}, {"Title"="", "Name"="", "Point"=0, "Plot"=FALSE, "Trend"=FALSE, "Cycle"=FALSE, "Field"=0, "Row On (Save Data)"=FALSE, "Group"=0}, {"Title"="", "Name"="", "Point"=0, "Plot"=FALSE, "Trend"=FALSE, "Cycle"=FALSE, "Field"=0, "Row On (Save Data)"=FALSE, "Group"=0}, {"Title"="", "Name"="", "Point"=0, "Plot"=FALSE, "Trend"=FALSE, "Cycle"=FALSE, "Field"=0, "Row On (Save Data)"=FALSE, "Group"=0}, {"Title"="", "Name"="", "Point"=0, "Plot"=FALSE, "Trend"=FALSE, "Cycle"=FALSE, "Field"=0, "Row On (Save Data)"=FALSE, "Group"=0}, {"Title"="", "Name"="", "Point"=0, "Plot"=FALSE, "Trend"=FALSE, "Cycle"=FALSE, "Field"=0, "Row On (Save Data)"=FALSE, "Group"=0}, {"Title"="", "Name"="", "Point"=0, "Plot"=FALSE, "Trend"=FALSE, "Cycle"=FALSE, "Field"=0, "Row On (Save Data)"=FALSE, "Group"=0}, {"Title"="", "Name"="", "Point"=0, "Plot"=FALSE, "Trend"=FALSE, "Cycle"=FALSE, "Field"=0, "Row On (Save Data)"=FALSE, "Group"=0}, {"Title"="", "Name"="", "Point"=0, "Plot"=FALSE, "Trend"=FALSE, "Cycle"=FALSE, "Field"=0, "Row On (Save Data)"=FALSE, "Group"=0}, {"Title"="", "Name"="", "Point"=0, "Plot"=FALSE, "Trend"=FALSE, "Cycle"=FALSE, "Field"=0, "Row On (Save Data)"=FALSE, "Group"=0}, {"Title"="", "Name"="", "Point"=0, "Plot"=FALSE, "Trend"=FALSE, "Cycle"=FALSE, "Field"=0, "Row On (Save Data)"=FALSE, "Group"=0}, {"Title"="", "Name"="", "Point"=0, "Plot"=FALSE, "Trend"=FALSE, "Cycle"=FALSE, "Field"=0, "Row On (Save Data)"=FALSE, "Group"=0}, {"Title"="", "Name"="", "Point"=0, "Plot"=FALSE, "Trend"=FALSE, "Cycle"=FALSE, "Field"=0, "Row On (Save Data)"=FALSE, "Group"=0}, {"Title"="", "Name"="", "Point"=0, "Plot"=FALSE, "Trend"=FALSE, "Cycle"=FALSE, "Field"=0, "Row On (Save Data)"=FALSE, "Group"=0}, {"Title"="", "Name"="", "Point"=0, "Plot"=FALSE, "Trend"=FALSE, "Cycle"=FALSE, "Field"=0, "Row On (Save Data)"=FALSE, "Group"=0}, {"Title"="", "Name"="", "Point"=0, "Plot"=FALSE, "Trend"=FALSE, "Cycle"=FALSE, "Field"=0, "Row On (Save Data)"=FALSE, "Group"=0}, {"Title"="", "Name"="", "Point"=0, "Plot"=FALSE, "Trend"=FALSE, "Cycle"=FALSE, "Field"=0, "Row On (Save Data)"=FALSE, "Group"=0}, {"Title"="", "Name"="", "Point"=0, "Plot"=FALSE, "Trend"=FALSE, "Cycle"=FALSE, "Field"=0, "Row On (Save Data)"=FALSE, "Group"=0}, {"Title"="", "Name"="", "Point"=0, "Plot"=FALSE, "Trend"=FALSE, "Cycle"=FALSE, "Field"=0, "Row On (Save Data)"=FALSE, "Group"=0}, {"Title"="", "Name"="", "Point"=0, "Plot"=FALSE, "Trend"=FALSE, "Cycle"=FALSE, "Field"=0, "Row On (Save Data)"=FALSE, "Group"=0}, {"Title"="", "Name"="", "Point"=0, "Plot"=FALSE, "Trend"=FALSE, "Cycle"=FALSE, "Field"=0, "Row On (Save Data)"=FALSE, "Group"=0}, {"Title"="", "Name"="", "Point"=0, "Plot"=FALSE, "Trend"=FALSE, "Cycle"=FALSE, "Field"=0, "Row On (Save Data)"=FALSE, "Group"=0}, {"Title"="", "Name"="", "Point"=0, "Plot"=FALSE, "Trend"=FALSE, "Cycle"=FALSE, "Field"=0, "Row On (Save Data)"=FALSE, "Group"=0}, {"Title"="", "Name"="", "Point"=0, "Plot"=FALSE, "Trend"=FALSE, "Cycle"=FALSE, "Field"=0, "Row On (Save Data)"=FALSE, "Group"=0}, {"Title"="", "Name"="", "Point"=0, "Plot"=FALSE, "Trend"=FALSE, "Cycle"=FALSE, "Field"=0, "Row On (Save Data)"=FALSE, "Group"=0}, {"Title"="", "Name"="", "Point"=0, "Plot"=FALSE, "Trend"=FALSE, "Cycle"=FALSE, "Field"=0, "Row On (Save Data)"=FALSE, "Group"=0}, {"Title"="", "Name"="", "Point"=0, "Plot"=FALSE, "Trend"=FALSE, "Cycle"=FALSE, "Field"=0, "Row On (Save Data)"=FALSE, "Group"=0}, {"Title"="", "Name"="", "Point"=0, "Plot"=FALSE, "Trend"=FALSE, "Cycle"=FALSE, "Field"=0, "Row On (Save Data)"=FALSE, "Group"=0}, {"Title"="", "Name"="", "Point"=0, "Plot"=FALSE, "Trend"=FALSE, "Cycle"=FALSE, "Field"=0, "Row On (Save Data)"=FALSE, "Group"=0}, {"Title"="", "Name"="", "Point"=0, "Plot"=FALSE, "Trend"=FALSE, "Cycle"=FALSE, "Field"=0, "Row On (Save Data)"=FALSE, "Group"=0}, {"Title"="", "Name"="", "Point"=0, "Plot"=FALSE, "Trend"=FALSE, "Cycle"=FALSE, "Field"=0, "Row On (Save Data)"=FALSE, "Group"=0}, {"Title"="", "Name"="", "Point"=0, "Plot"=FALSE, "Trend"=FALSE, "Cycle"=FALSE, "Field"=0, "Row On (Save Data)"=FALSE, "Group"=0}, {"Title"="", "Name"="", "Point"=0, "Plot"=FALSE, "Trend"=FALSE, "Cycle"=FALSE, "Field"=0, "Row On (Save Data)"=FALSE, "Group"=0}, {"Title"="", "Name"="", "Point"=0, "Plot"=FALSE, "Trend"=FALSE, "Cycle"=FALSE, "Field"=0, "Row On (Save Data)"=FALSE, "Group"=0}, {"Title"="", "Name"="", "Point"=0, "Plot"=FALSE, "Trend"=FALSE, "Cycle"=FALSE, "Field"=0, "Row On (Save Data)"=FALSE, "Group"=0}, {"Title"="", "Name"="", "Point"=0, "Plot"=FALSE, "Trend"=FALSE, "Cycle"=FALSE, "Field"=0, "Row On (Save Data)"=FALSE, "Group"=0}, {"Title"="", "Name"="", "Point"=0, "Plot"=FALSE, "Trend"=FALSE, "Cycle"=FALSE, "Field"=0, "Row On (Save Data)"=FALSE, "Group"=0}, {"Title"="", "Name"="", "Point"=0, "Plot"=FALSE, "Trend"=FALSE, "Cycle"=FALSE, "Field"=0, "Row On (Save Data)"=FALSE, "Group"=0}, {"Title"="", "Name"="", "Point"=0, "Plot"=FALSE, "Trend"=FALSE, "Cycle"=FALSE, "Field"=0, "Row On (Save Data)"=FALSE, "Group"=0}, {"Title"="", "Name"="", "Point"=0, "Plot"=FALSE, "Trend"=FALSE, "Cycle"=FALSE, "Field"=0, "Row On (Save Data)"=FALSE, "Group"=0}, {"Title"="", "Name"="", "Point"=0, "Plot"=FALSE, "Trend"=FALSE, "Cycle"=FALSE, "Field"=0, "Row On (Save Data)"=FALSE, "Group"=0}, {"Title"="", "Name"="", "Point"=0, "Plot"=FALSE, "Trend"=FALSE, "Cycle"=FALSE, "Field"=0, "Row On (Save Data)"=FALSE, "Group"=0}, {"Title"="", "Name"="", "Point"=0, "Plot"=FALSE, "Trend"=FALSE, "Cycle"=FALSE, "Field"=0, "Row On (Save Data)"=FALSE, "Group"=0}, {"Title"="", "Name"="", "Point"=0, "Plot"=FALSE, "Trend"=FALSE, "Cycle"=FALSE, "Field"=0, "Row On (Save Data)"=FALSE, "Group"=0}, {"Title"="", "Name"="", "Point"=0, "Plot"=FALSE, "Trend"=FALSE, "Cycle"=FALSE, "Field"=0, "Row On (Save Data)"=FALSE, "Group"=0}, {"Title"="", "Name"="", "Point"=0, "Plot"=FALSE, "Trend"=FALSE, "Cycle"=FALSE, "Field"=0, "Row On (Save Data)"=FALSE, "Group"=0}, {"Title"="", "Name"="", "Point"=0, "Plot"=FALSE, "Trend"=FALSE, "Cycle"=FALSE, "Field"=0, "Row On (Save Data)"=FALSE, "Group"=0}, {"Title"="", "Name"="", "Point"=0, "Plot"=FALSE, "Trend"=FALSE, "Cycle"=FALSE, "Field"=0, "Row On (Save Data)"=FALSE, "Group"=0}, {"Title"="", "Name"="", "Point"=0, "Plot"=FALSE, "Trend"=FALSE, "Cycle"=FALSE, "Field"=0, "Row On (Save Data)"=FALSE, "Group"=0}, {"Title"="", "Name"="", "Point"=0, "Plot"=FALSE, "Trend"=FALSE, "Cycle"=FALSE, "Field"=0, "Row On (Save Data)"=FALSE, "Group"=0}, {"Title"="", "Name"="", "Point"=0, "Plot"=FALSE, "Trend"=FALSE, "Cycle"=FALSE, "Field"=0, "Row On (Save Data)"=FALSE, "Group"=0}, {"Title"="", "Name"="", "Point"=0, "Plot"=FALSE, "Trend"=FALSE, "Cycle"=FALSE, "Field"=0, "Row On (Save Data)"=FALSE, "Group"=0}, {"Title"="", "Name"="", "Point"=0, "Plot"=FALSE, "Trend"=FALSE, "Cycle"=FALSE, "Field"=0, "Row On (Save Data)"=FALSE, "Group"=0}, {"Title"="", "Name"="", "Point"=0, "Plot"=FALSE, "Trend"=FALSE, "Cycle"=FALSE, "Field"=0, "Row On (Save Data)"=FALSE, "Group"=0}, {"Title"="", "Name"="", "Point"=0, "Plot"=FALSE, "Trend"=FALSE, "Cycle"=FALSE, "Field"=0, "Row On (Save Data)"=FALSE, "Group"=0}, {"Title"="", "Name"="", "Point"=0, "Plot"=FALSE, "Trend"=FALSE, "Cycle"=FALSE, "Field"=0, "Row On (Save Data)"=FALSE, "Group"=0}, {"Title"="", "Name"="", "Point"=0, "Plot"=FALSE, "Trend"=FALSE, "Cycle"=FALSE, "Field"=0, "Row On (Save Data)"=FALSE, "Group"=0}, {"Title"="", "Name"="", "Point"=0, "Plot"=FALSE, "Trend"=FALSE, "Cycle"=FALSE, "Field"=0, "Row On (Save Data)"=FALSE, "Group"=0}, {"Title"="", "Name"="", "Point"=0, "Plot"=FALSE, "Trend"=FALSE, "Cycle"=FALSE, "Field"=0, "Row On (Save Data)"=FALSE, "Group"=0}, {"Title"="", "Name"="", "Point"=0, "Plot"=FALSE, "Trend"=FALSE, "Cycle"=FALSE, "Field"=0, "Row On (Save Data)"=FALSE, "Group"=0}, {"Title"="", "Name"="", "Point"=0, "Plot"=FALSE, "Trend"=FALSE, "Cycle"=FALSE, "Field"=0, "Row On (Save Data)"=FALSE, "Group"=0}, {"Title"="", "Name"="", "Point"=0, "Plot"=FALSE, "Trend"=FALSE, "Cycle"=FALSE, "Field"=0, "Row On (Save Data)"=FALSE, "Group"=0}, {"Title"="", "Name"="", "Point"=0, "Plot"=FALSE, "Trend"=FALSE, "Cycle"=FALSE, "Field"=0, "Row On (Save Data)"=FALSE, "Group"=0}, {"Title"="", "Name"="", "Point"=0, "Plot"=FALSE, "Trend"=FALSE, "Cycle"=FALSE, "Field"=0, "Row On (Save Data)"=FALSE, "Group"=0}, {"Title"="", "Name"="", "Point"=0, "Plot"=FALSE, "Trend"=FALSE, "Cycle"=FALSE, "Field"=0, "Row On (Save Data)"=FALSE, "Group"=0}, {"Title"="", "Name"="", "Point"=0, "Plot"=FALSE, "Trend"=FALSE, "Cycle"=FALSE, "Field"=0, "Row On (Save Data)"=FALSE, "Group"=0}, {"Title"="", "Name"="", "Point"=0, "Plot"=FALSE, "Trend"=FALSE, "Cycle"=FALSE, "Field"=0, "Row On (Save Data)"=FALSE, "Group"=0}, {"Title"="", "Name"="", "Point"=0, "Plot"=FALSE, "Trend"=FALSE, "Cycle"=FALSE, "Field"=0, "Row On (Save Data)"=FALSE, "Group"=0}]  # Point Array
        w214 = T7 {"Current VI Reference"=refnum, "Close Panel on Exit?"=FALSE}  # Core
        w215 = FALSE  # Default Headers
        n84 = Build Path(base path="Tool Base Path", name or relative path="Point") -> (appended path=w210:path)
        n85 = Bundle("Core"=w214, "Default Headers"=w215, "Header Save Array"="Header Save Array", "Chamber Data"="Chamber Data", "appended path"=w210, "Point Array"=w209, "Write Path"=w208, "Tree Selection"="Tree Selection", "Point Startup (WasherDOE)"="Point Startup (WasherDOE)") -> (w217:T6)  [unwired: 1 in]
        n86 = call <vilib>:"Add State(s) to Queue__jki_lib_state_machine.vi"("State(s) in (\"\")"=w219) -> ("States Out"=w218:string)  [unwired: 14 in]
      }
      frame "Data: Cleanup" {
        # "Cleanup any data and references, here.\n(this is called automatically, by the Macro: Exit)"
        n87 = Unbundle By Name(w220) -> ("Core.Current VI Reference"=w223:refnum<vi>)
        n88 = Close Reference(reference=w223, error in (no error)=w222) -> (error out=w221:errorcluster)
        n89 = call <vilib>:"Add State(s) to Queue__jki_lib_state_machine.vi"("State(s) in (\"\")"=w225) -> ("States Out"=w224:string)  [unwired: 14 in]
      }
      frame "---------- UI ----------" {
        # "Do not put any code in this frame.\n(It is a separator no-op. You can make a copy of this frame to create a new UI frame)"
        n90 = call <vilib>:"Add State(s) to Queue__jki_lib_state_machine.vi"("State(s) in (\"\")"=w229) -> ("States Out"=w228:string)  [unwired: 14 in]
      }
      frame "UI: Initialize" {
        w233 = FALSE  # Old?
        n91 = case shown="False" w233 {
          tunnel: w235 -> [w243 w268]
          tunnel: [w243 w267] -> w234
          tunnel: w232 -> [w253 w266]
          tunnel: [w246 w266] -> w231
          tunnel: [w250 ""] -> w230
          frame False {
            n92 = Unbundle By Name(w243) -> ("Point Startup (WasherDOE)"=w238:path, "appended path"=w252:path, "Tree Selection"=w245:T2, "Chamber Data"=w244:string[][])
            n93 = Equal?(x=path "", y=w238) -> (x = y?=w239:bool)
            n94 = call "UTILITY Get Point File List.vi"("error in (no error)"=w253, "Folder Path"=w252) -> ("error out"=w247:errorcluster, "Point File Names"=w251:string[])  [unwired: 8 in]
            n95 = property on="Point File Name" class="CmbBox"("Strings[]"=w251) -> ()  [unwired: 2 in, 2 out]
            n96 = call "RTS Extract Point Array.vi"("Error In"=w247, "Chamber Data in"=w244, "Tree Selection in"=w245) -> ("Error Out"=w249:errorcluster, "Chamber Data out"=w248:string[][])  [unwired: 7 in]
            n97 = call "RTS Get Point Location.vi"("Error In"=w249, "Full List Box Data"=w248) -> ("Error Out"=w246:errorcluster, "Point File Name"=w242:string)  [unwired: 7 in, 1 out]
            n98 = case shown="True" w239 {
              tunnel: ["Read Point File" w261] -> w250
              tunnel: w242 -> [_ w258]
              tunnel: [w254 w257] -> w241
              tunnel: w238 -> [w255 _]
              frame False {
                # "I use this in Washer DOE"
                n99 = call <vilib>:"Get File Extension.vi"("file"=w255) -> ("filename without extension"=w254:string)  [unwired: 6 in, 4 out]
              }
              frame True {
                n100 = Equal?(x="Configure Point File", y=w258) -> (x = y?=w259:bool)
                n101 = case shown="True" w259 {
                  tunnel: ["Read Point File" w264] -> w261
                  tunnel: w258 -> [w262 _]
                  tunnel: [w262 w264] -> w257
                  frame False {
                  }
                  frame True {
                    w264 = ""
                  }
                }
              }
            }
            n102 = local write "Point File Name"(w241) -> ()
          }
          frame True {
            n103 = Unbundle By Name(w268) -> ("appended path"=w272:path, "Chamber Data"=w270:string[][])
            n104 = call "Dynamic Headers Read Header File.vi"("Read/Write (True/False)"=TRUE, "Save Data (READ ONLY)"=w270, "Tool Base Path"=w272) -> ("New Header Save Array (READ ONLY)"=w271:T1[])  [unwired: 7 in, 1 out]
            n105 = property on="Header Save Array" class="Arr (strict)"("Value"=w271) -> ()  [unwired: 2 in, 2 out]
            n106 = Bundle By Name(cluster=w268, "Header Save Array"=w271) -> (w267:T6)
          }
        }
        n107 = call <vilib>:"Add State(s) to Queue__jki_lib_state_machine.vi"("State(s) in Front (\"\")"=w230, "State(s) in (\"\")"=w237) -> ("States Out"=w236:string)  [unwired: 13 in]
      }
      frame "UI: Cursor Set" {
        # "Argument"
        # "Set and Unset Cursor Busy.\n(Usage: \"UI: Cursor Set >> Busy|Idle\")"
        n108 = case shown="\"Idle\", Default" w273 {
          tunnel: w275 -> [w280 w282]
          tunnel: [w279 w281] -> w274
          frame "Idle", Default {
            n109 = call <vilib>:"Unset Busy.vi"("error in (no error)"=w280) -> ("error out"=w279:errorcluster)  [unwired: 10 in]
          }
          frame "Busy" {
            n110 = call <vilib>:"Set Busy.vi"("error in (no error)"=w282) -> ("error out"=w281:errorcluster)  [unwired: 9 in, 1 out]
          }
        }
        n111 = call <vilib>:"Add State(s) to Queue__jki_lib_state_machine.vi"("State(s) in (\"\")"=w278) -> ("States Out"=w277:string)  [unwired: 14 in]
      }
      frame "UI: Front Panel State" {
        # "Argument"
        # "Set Front Panel Open or Closed\n(Usage: \"UI: Front Panel State >> Open|Close\")"
        n112 = Unbundle By Name(w285) -> ("Core.Current VI Reference"=w284:refnum<vi>)
        n113 = case shown="\"Open\", Default" w283 {
          tunnel: w287 -> [w293 w306]
          tunnel: [w295 w307] -> w286
          tunnel: w284 -> [w294 w304]
          frame "Open", Default {
            n114 = property class="VI"(reference=w294, error in=w293) -> (reference out=w291:refnum<vi>, error out=w292:errorcluster, "Front Panel.Open"=w290:bool)
            n115 = case shown="False" w290 {
              tunnel: [w298 w301] -> w295
              tunnel: w292 -> [w297 w301]
              tunnel: w291 -> [w296 _]
              frame False {
                n116 = invoke class="VI" method="FP.Open"(reference=w296, error in=w297, "Activate"=TRUE, "State"=T5."Standard") -> (error out=w298:errorcluster)  [unwired: 1 in, 4 out]
              }
              frame True {
              }
            }
          }
          frame "Close" {
            n117 = property class="VI"(reference=w304, error in=w306) -> (reference out=w303:refnum<vi>, error out=w305:errorcluster, "Front Panel.Open"=w302:bool)
            n118 = case shown="True" w302 {
              tunnel: [w308 w311] -> w307
              tunnel: w305 -> [w308 w310]
              tunnel: w303 -> [_ w309]
              frame False {
              }
              frame True {
                n119 = invoke class="VI" method="FP.Close"(reference=w309, error in=w310) -> (error out=w311:errorcluster)  [unwired: 1 in, 2 out]
              }
            }
          }
        }
        n120 = call <vilib>:"Add State(s) to Queue__jki_lib_state_machine.vi"("State(s) in (\"\")"=w289) -> ("States Out"=w288:string)  [unwired: 14 in]
      }
      frame "---------- Macro ----------" {
        # "Do not put any code in this frame.\n(It is a separator no-op. You can make a copy of this frame to create a new Macro frame)"
        n121 = call <vilib>:"Add State(s) to Queue__jki_lib_state_machine.vi"("State(s) in (\"\")"=w315) -> ("States Out"=w314:string)  [unwired: 14 in]
      }
      frame "Macro: Initialize" {
        w316 = "Data: Initialize\nInitialize Core Data\nUI: Initialize\nUI: Front Panel State >> Open"  # Data: Initialize Initialize Core Data UI: Initialize UI: Front Panel State >> Open
        n122 = call <vilib>:"Add State(s) to Queue__jki_lib_state_machine.vi"("State(s) in Front (\"\")"=w316, "State(s) in (\"\")"=w320) -> ("States Out"=w319:string)  [unwired: 13 in]
      }
      frame "Read Point File" {
        n123 = Unbundle By Name(w333) -> ("Point Array"=w324:T3[], "Tree Selection"=w325:T2, "Chamber Data"=w326:string[][], "appended path"=w338:path)
        n124 = Concatenate Strings("Point File Name", ".Pnt" ("pattern")) -> (w327:string)
        n125 = Build Path(base path=w338, name or relative path=w327) -> (appended path=w330:path)
        n126 = call "RTS Read Point File.vi"("Error In"=w337, "Path"=w330) -> ("Error Out"=w335:errorcluster, "Point File"=w322:T3[])  [unwired: 7 in, 1 out]
        n127 = Replace Array Subset(array=w324, new element=w322, index=0) -> (w321:T3[])
        "Point Data" <- w321
        n128 = call "Dynamic Headers Read Header File.vi"("Tree Selection"=w325, "Read/Write (True/False)"=TRUE, "Error In"=w335, "Point Data"=w322, "Save Data (READ ONLY)"=w326, "Tool Base Path"=w330) -> ("Error Out"=w334:errorcluster, "New Header Save Array (READ ONLY)"=w331:T1[])  [unwired: 4 in]
        n129 = Bundle By Name(cluster=w333, "Point Array"=w321, "Header Save Array"=w331) -> (w332:T6)
        n130 = local write "Header Save Array"(w331) -> ()
        n131 = call <vilib>:"Add State(s) to Queue__jki_lib_state_machine.vi"("State(s) in (\"\")"=w340) -> ("States Out"=w339:string)  [unwired: 14 in]
      }
      frame "Write Point File" {
        # "It seems that the Point Array does not\nkeep track of the changes made to the \nlast line of the \"Change Header\" VI while \nthe Header Save Array does keep track of\nthe changes. 10/25/18"
        n132 = Unbundle By Name(w348) -> ("appended path"=w341:path, "Write Path"=w346:path, "Point Array"=w347:T3[], "Header Save Array"=w345:T1[])
        n133 = call "RTS Write Point File.vi"("Error In"=w349, "Header Save Array Input"=w345, "Point Data"=w347, "Path"=w346) -> ("Error Out"=w343:errorcluster)  [unwired: 7 in]
        n134 = call "UTILITY Get Point File List.vi"("error in (no error)"=w343, "Folder Path"=w341) -> ("error out"=w342:errorcluster, "Point File Names"=w344:string[])  [unwired: 8 in]
        n135 = property on="Point File Name" class="CmbBox"("Strings[]"=w344) -> ()  [unwired: 2 in, 2 out]
        n136 = call <vilib>:"Add State(s) to Queue__jki_lib_state_machine.vi"("State(s) in (\"\")"=w351) -> ("States Out"=w350:string)  [unwired: 14 in]
      }
      frame "Delete Point File" {
        # "When you delete a file..update the \ndrop down list"
        n137 = local read "Point File Name"() -> (w362:string)
        n138 = Unbundle By Name(w364) -> ("appended path"=w354:path)
        n139 = Concatenate Strings(w362, ".Pnt" ("pattern")) -> (w361:string)
        n140 = Build Path(base path=w354, name or relative path=w361) -> (appended path=w360:path)
        n141 = call <vilib>:"Check if File or Folder Exists.vi"("error in (no error)"=w359, "path"=w360) -> ("error out"=w357:errorcluster, "dup path"=w358:path)  [unwired: 7 in, 1 out]
        n142 = Delete(path (use dialog)=w358, error in=w357) -> (error out=w355:errorcluster)  [unwired: 3 in, 2 out]
        n143 = call "UTILITY Get Point File List.vi"("error in (no error)"=w355, "Folder Path"=w354) -> ("error out"=w353:errorcluster, "Point File Names"=w356:string[])  [unwired: 8 in]
        n144 = flat-sequence {
          tunnel: w353 -> [w368]
          tunnel: [w368] -> w352
          frame #0 {
            n145 = local write "Point File Name"("") -> ()
          }
        }
        n146 = property on="Point File Name" class="CmbBox"("Strings[]"=w356) -> ()  [unwired: 2 in, 2 out]
        n147 = call <vilib>:"Add State(s) to Queue__jki_lib_state_machine.vi"("State(s) in (\"\")"=w366) -> ("States Out"=w365:string)  [unwired: 14 in]
      }
      frame "Macro: Exit" {
        # "Exit Macro\n(This is called once, when the VI exits)"
        n148 = Unbundle By Name(w375) -> ("Core.Close Panel on Exit?"=w374:bool)
        n149 = Select(t="UI: Front Panel State >> Close", s=w374, f="") -> (s? t:f=w371:string)
        n150 = call <vilib>:"Add State(s) to Queue__jki_lib_state_machine.vi"("State(s) in (\"\")"=w371, "State(s) at Back (\"\")"="Data: Cleanup\nExit") -> ("States Out"=w369:string)  [unwired: 13 in]
        n151 = call <vilib>:"Add State(s) to Queue__jki_lib_state_machine.vi"("State(s) in Front (\"\")"=w369, "State(s) in (\"\")"=w378) -> ("States Out"=w377:string)  [unwired: 13 in]
      }
    }
    n152 = case shown="True" "Debug" {
      tunnel: w19 -> [w30 w33]
      tunnel: w18 -> [_ w32]
      tunnel: [w30 w31] -> w17
      frame False {
      }
      frame True {
        n153 = Build Array (concatenate)(w33, w32) -> (w31:string[])
      }
    }
    "Debug States" <- w17
  }
  "Error Out" <- w8
  n154 = Unbundle By Name(w3) -> ("Write Path"=→"Point File Path":path, "Default Headers"=→"Default Headers":bool)
